vi "RefData(SubVI).vi"() -> (0 "Events":dbl format="%0.2f")   [LabVIEW 2013, in "main.lvlib"]
uses:
  main.lvlib
  Controls/Enum User Events.ctl
  <vilib>/DAQmx/read.llb/DAQmx Read (Counter DBL 1Chan 1Samp).vi
  <vilib>/DAQmx/create/channels.llb/DAQmx Create Channel (CI-Count Edges).vi
  <vilib>/DAQmx/miscellaneous.llb/DAQmx Fill In Error Info.vi
panel:
  in  "Idle":bool
  in  "Start":bool=TRUE
  in  "Stop":bool=TRUE
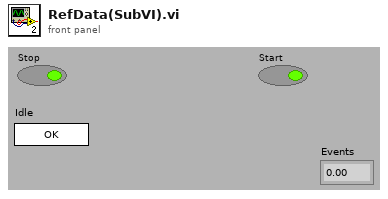
[diagram p1: front panel]
types:
  T1 = typedef "main.lvlib/Enum User Events.ctl" = enum16{"User Event", "Init"}
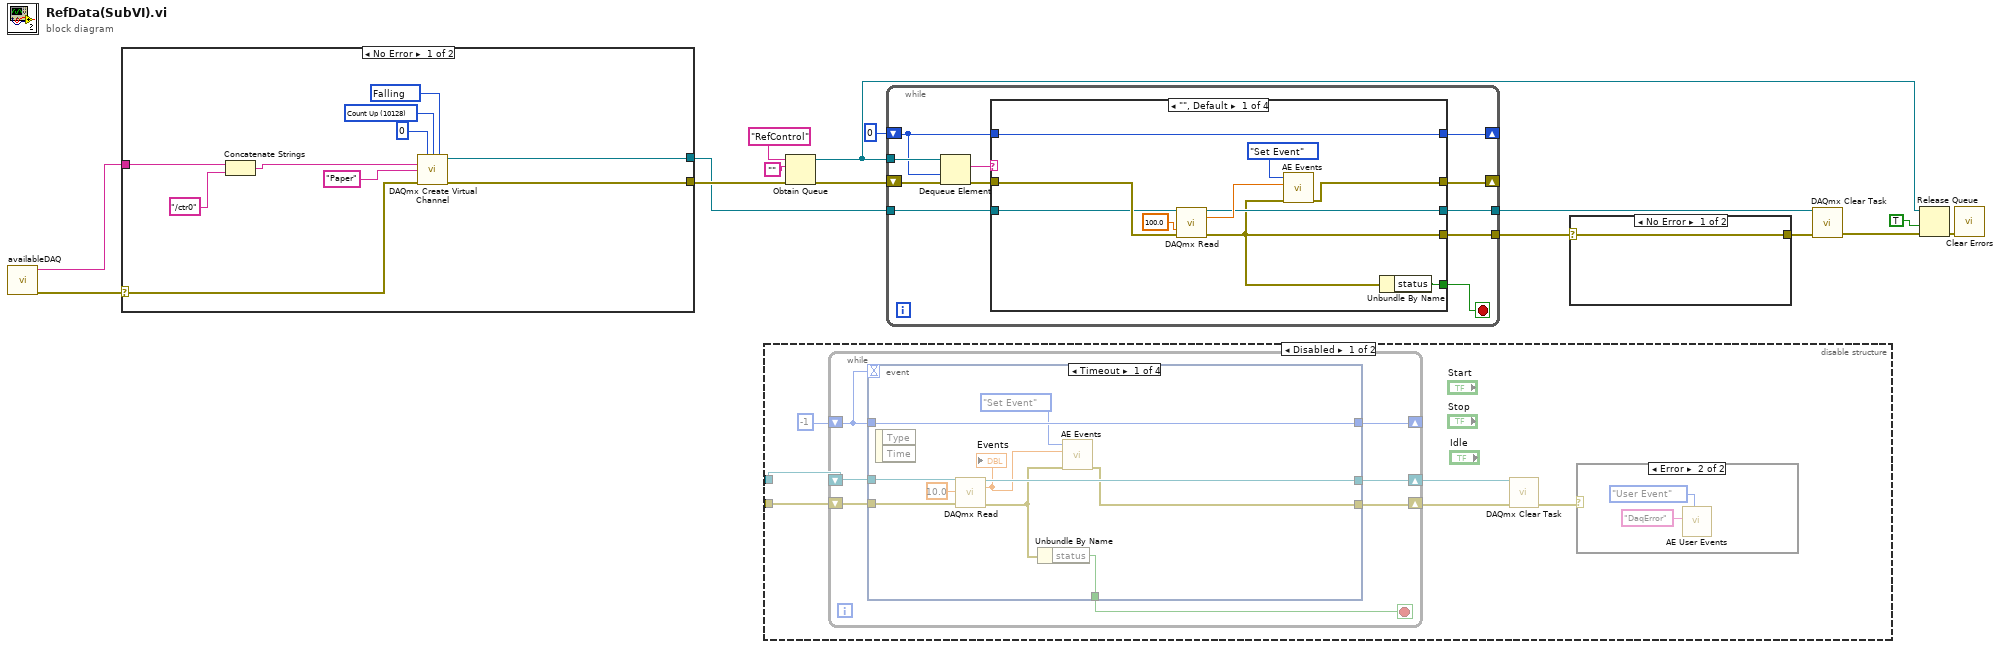
[diagram p0: block diagram]
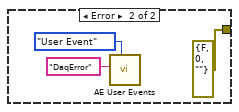
[diagram p2: hidden frame]
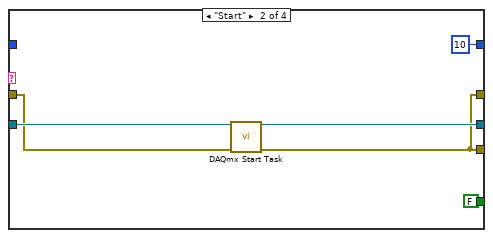
[diagram p3: hidden frame]
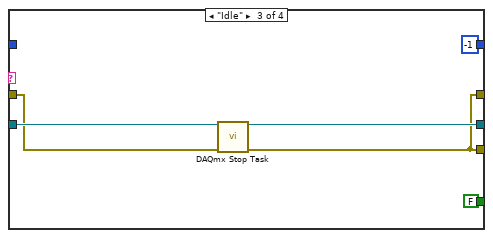
[diagram p4: hidden frame]
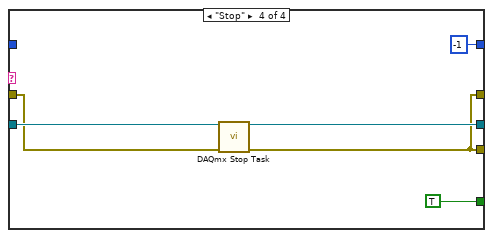
[diagram p5: hidden frame]
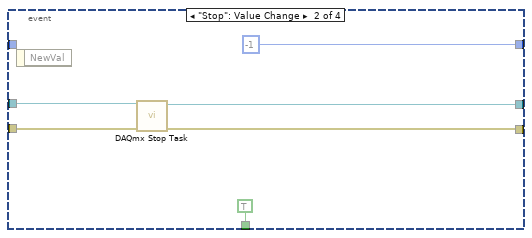
[diagram p7: hidden frame]
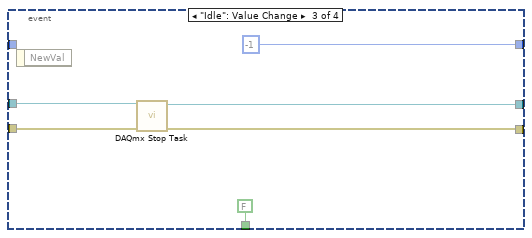
[diagram p8: hidden frame]
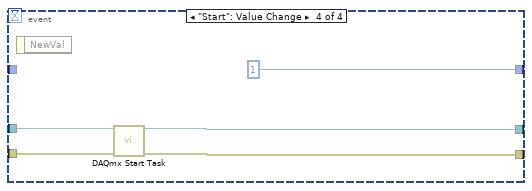
[diagram p9: hidden frame]
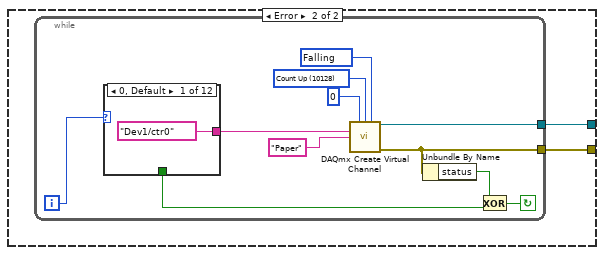
[diagram p11: hidden frame]
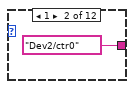
[diagram p12: hidden frame]
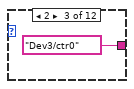
[diagram p13: hidden frame]
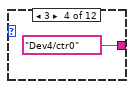
[diagram p14: hidden frame]
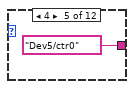
[diagram p15: hidden frame]
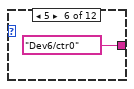
[diagram p16: hidden frame]
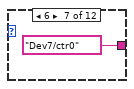
[diagram p17: hidden frame]
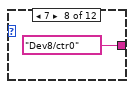
[diagram p18: hidden frame]
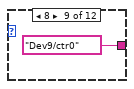
[diagram p19: hidden frame]
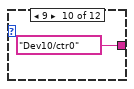
[diagram p20: hidden frame]
diagram:
  n1 = call "availableDAQ.vi"() -> ("error out"=w15:errorcluster, "DAQmx Device Name"=w14:tag)  [unwired: 10 in]
  n2 = case shown="No Error" w15 {
    selector: w15 -> [w16 _]
    tunnel: [w20 w27] -> w1
    tunnel: [w21 w26] -> w13
    tunnel: w14 -> [w19 _]
    frame No Error {
      w23 = 10128 items=["Count Up"=10128, "Count Down"=10124, "Externally Controlled"=10326] ("count direction")
      w24 = 10171 items=["Rising"=10280, "Falling"=10171] ("edge")
      n3 = Concatenate Strings(w19, "/ctr0") -> (w17:string)
      n4 = call-poly <vilib>:"DAQmx Create Virtual Channel.vi"("initial count"=u32 0, "count direction"=w23, "edge"=w24, "counter"=w17, "name to assign"="Paper", "error in"=w16) -> ("task out"=w20:refnum<k21>, "error out"=w21:errorcluster)  [unwired: 8 in]
    }
    frame Error {
      n5 = while {
        tunnel: [w33] -> w27
        tunnel: [w31] -> w26
        i -> [w32]
        stop <- w30 continue-if-true
        w36 = 10128 items=["Count Up"=10128, "Count Down"=10124, "Externally Controlled"=10326] ("count direction")
        w37 = 10171 items=["Rising"=10280, "Falling"=10171] ("edge")
        n6 = case shown="0, Default" w32 {
          tunnel: [tag "Dev1/ctr0" ("lines") tag "Dev2/ctr0" ("lines") tag "Dev3/ctr0" ("lines") tag "Dev4/ctr0" ("lines") tag "Dev5/ctr0" ("lines") tag "Dev6/ctr0" ("lines") tag "Dev7/ctr0" ("lines") tag "Dev8/ctr0" ("lines") tag "Dev9/ctr0" ("lines") tag "Dev10/ctr0" ("lines") tag "Dev11/ctr0" ("lines") tag "" ("lines")] -> w34
          tunnel: [_ _ _ _ _ _ _ _ _ _ _ TRUE] -> w28
          frame 0, Default {
          }
          frame 1 {
          }
          frame 2 {
          }
          frame 3 {
          }
          frame 4 {
          }
          frame 5 {
          }
          frame 6 {
          }
          frame 7 {
          }
          frame 8 {
          }
          frame 9 {
          }
          frame 10 {
          }
          frame 11 {
          }
        }
        n7 = call-poly <vilib>:"DAQmx Create Virtual Channel.vi"("initial count"=u32 0, "count direction"=w36, "edge"=w37, "counter"=w34, "name to assign"="Paper") -> ("task out"=w33:refnum<k21>, "error out"=w31:errorcluster)  [unwired: 9 in]
        n8 = Unbundle By Name(w31) -> ("status"=w29:bool)
        n9 = Exclusive Or(1:w28, 2:w29) -> (0:w30:bool)
      }
    }
  }
  n10 = disable-structure shown="Disabled" {
    disable-tunnel: _ -> [w54 _]
    disable-tunnel: _ -> [w53 _]
    frame Disabled {
      n11 = while {
        shift-right: [w62] -> _
        shift-left: -1 -> [w61]
        shift-right: [w64] -> w56
        shift-left: w54 -> [w66]
        shift-right: [w63] -> w55
        shift-left: w53 -> [w65]
        stop <- w60 stop-if-true
        n12 = event shown="[0] Timeout" {
          selector: _ -> [_ _ _ _]
          dyn-events: _ -> [_ _ _ _]
          timeout: w61 -> [_ _ _ _]
          tunnel: w66 -> [w75 w81 w87 w89]
          tunnel: w65 -> [w74 w80 w86 w92]
          tunnel: [w73 w78 w84 w90] -> w64
          tunnel: [w67 w79 w85 w91] -> w63
          tunnel: [w72 -1 ("f") -1 ("f") 1 ("f")] -> w62
          tunnel: w61 -> [w72 _ _ _]
          tunnel: [w71 TRUE ("status") FALSE ("status") _] -> w60
          event Timeout {
            n13 = event-data() -> ()  [unwired: 1 in, 2 out]
            n14 = call-poly <vilib>:"DAQmx Read.vi"("task/channels in"=w75, "timeout"=10.0, "error in"=w74) -> ("task out"=w73:refnum<k21>, "data"=w70:dbl, "error out"=w68:errorcluster)  [unwired: 10 in]
            "Events" <- w70
            n15 = Unbundle By Name(w68) -> ("status"=w71:bool)
            n16 = call "AE Events.vi"("error in (no error)"=w68, "Event In"=w70, "Action"=enum16{"Init", "Get Event", "Set Event"}."Set Event") -> ("error out"=w67:errorcluster)  [unwired: 7 in, 1 out]
          }
          event "Stop": Value Change {
            n17 = event-data() -> ()  [unwired: 1 in, 1 out]
            n18 = call <vilib>:"DAQmx Stop Task.vi"("task/channels in"=w81, "error in"=w80) -> ("task out"=w78:refnum<k21>, "error out"=w79:errorcluster)  [unwired: 12 in]
          }
          event "Idle": Value Change {
            n19 = event-data() -> ()  [unwired: 1 in, 1 out]
            n20 = call <vilib>:"DAQmx Stop Task.vi"("task/channels in"=w87, "error in"=w86) -> ("task out"=w84:refnum<k21>, "error out"=w85:errorcluster)  [unwired: 12 in]
          }
          event "Start": Value Change {
            n21 = event-data() -> ()  [unwired: 1 in, 1 out]
            n22 = call <vilib>:"DAQmx Start Task.vi"("task/channels in"=w89, "error in"=w92) -> ("task out"=w90:refnum<k21>, "error out"=w91:errorcluster)  [unwired: 12 in]
          }
        }
      }
      n23 = call <vilib>:"DAQmx Clear Task.vi"("task in"=w56, "error in"=w55) -> ("error out"=w52:errorcluster)  [unwired: 13 in]
      n24 = case shown="Error" w52 {
        frame No Error {
        }
        frame Error {
          n25 = call "AE User Events.vi"("Action"=Enum_User_Events."User Event", "User Event"="DaqError") -> ()  [unwired: 8 in, 2 out]
        }
      }
    }
    frame Enabled {
    }
  }
  n26 = Obtain Queue(name (unnamed)="RefControl", element data type="", error in (no error)=w13) -> (queue out=w5:refnum<queue>, error out=w4:errorcluster)  [unwired: 2 in, 1 out]
  n27 = while {
    tunnel: w5 -> [w104]
    shift-right: [w101] -> _
    shift-left: w4 -> [w103]
    tunnel: w1 -> [w99]
    shift-right: [w96] -> _
    shift-left: 0 -> [w97]
    tunnel: [w95] -> w2
    tunnel: [w94] -> w3
    stop <- w98 stop-if-true
    n28 = Dequeue Element(queue=w104, timeout in ms (-1)=w97, error in (no error)=w103) -> (element=w102:string, error out=w100:errorcluster)  [unwired: 2 out]
    n29 = case shown="\"\", Default" w102 {
      tunnel: [w108 w115 w121 w127] -> w101
      tunnel: w100 -> [w112 w119 w125 w131]
      tunnel: w99 -> [w110 w120 w126 w132]
      tunnel: [w107 FALSE FALSE TRUE] -> w98
      tunnel: w97 -> [w111 _ _ _]
      tunnel: [w111 10 -1 -1] -> w96
      tunnel: [w106 w116 w122 w129] -> w95
      tunnel: [w105 w115 w121 w127] -> w94
      frame "", Default {
        n30 = call-poly <vilib>:"DAQmx Read.vi"("task/channels in"=w110, "timeout"=100.0, "error in"=w112) -> ("task out"=w106:refnum<k21>, "data"=w113:dbl, "error out"=w105:errorcluster)  [unwired: 10 in]
        n31 = call "AE Events.vi"("error in (no error)"=w105, "Event In"=w113, "Action"=enum16{"Init", "Get Event", "Set Event"}."Set Event") -> ("error out"=w108:errorcluster)  [unwired: 7 in, 1 out]
        n32 = Unbundle By Name(w105) -> ("status"=w107:bool)
      }
      frame "Start" {
        n33 = call <vilib>:"DAQmx Start Task.vi"("task/channels in"=w120, "error in"=w119) -> ("task out"=w116:refnum<k21>, "error out"=w115:errorcluster)  [unwired: 12 in]
      }
      frame "Idle" {
        n34 = call <vilib>:"DAQmx Stop Task.vi"("task/channels in"=w126, "error in"=w125) -> ("task out"=w122:refnum<k21>, "error out"=w121:errorcluster)  [unwired: 12 in]
      }
      frame "Stop" {
        n35 = call <vilib>:"DAQmx Stop Task.vi"("task/channels in"=w132, "error in"=w131) -> ("task out"=w129:refnum<k21>, "error out"=w127:errorcluster)  [unwired: 12 in]
      }
    }
  }
  n36 = case shown="No Error" w3 {
    selector: w3 -> [w133 _]
    tunnel: [w133 errorcluster {"status"=FALSE, "code"=0, "source"=""} ("error IO")] -> w8
    frame No Error {
    }
    frame Error {
      n37 = call "AE User Events.vi"("Action"=Enum_User_Events."User Event", "User Event"="DaqError") -> ()  [unwired: 8 in, 2 out]
    }
  }
  n38 = call <vilib>:"DAQmx Clear Task.vi"("task in"=w2, "error in"=w8) -> ("error out"=w7:errorcluster)  [unwired: 13 in]
  n39 = Release Queue(queue=w5, force destroy? (F)=TRUE, error in (no error)=w7) -> (error out=w6:errorcluster)  [unwired: 2 out]
  n40 = call <vilib>:"Clear Errors.vi"("error in (no error)"=w6) -> ()  [unwired: 6 in, 1 out]
